vi "Open vi Reference_3.0.0.0.vi"(4 "Close Front Panel(T)":bool, 5 "Wait Until Done":bool=TRUE, 6 "Front Panel State":T1(ring)=enum."Standard", 7 "Auto Dispose Reference":bool, 8 "error in":errorcluster, 10 "vi path":path) -> (0 "error out":errorcluster, 2 "vi reference":refnum<vi>, 3 "hist_rev":string)   [LabVIEW 2018]
uses:
  <vilib>/Utility/error.llb/DialogType.ctl
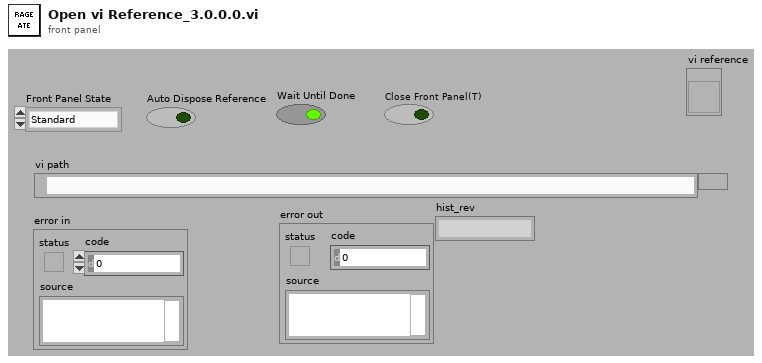
[diagram p1: front panel]
types:
  T1 = enum32{"Invalid", "Standard", "Closed", "Hidden", "Minimized", "Maximized"}
  T2 = typedef "DialogType.ctl" = u16
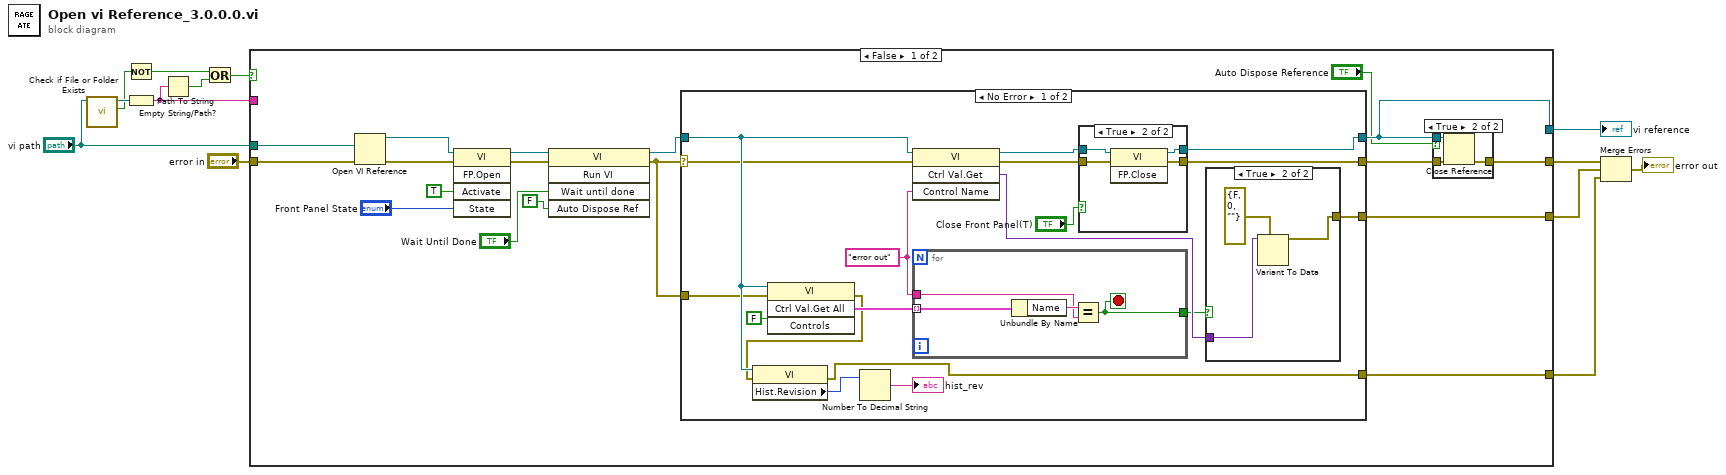
[diagram p0: block diagram]
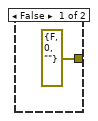
[diagram p3: hidden frame]
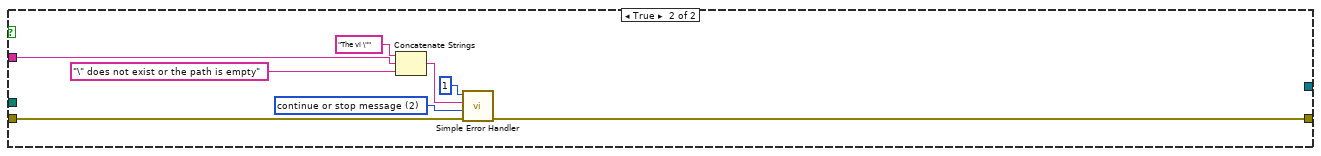
[diagram p6: hidden frame]
diagram:
  n1 = call <vilib>:"Check if File or Folder Exists.vi"("path"="vi path") -> ("file or folder exists?"=w8:bool, "dup path"=w10:path)  [unwired: 8 in, 1 out]
  n2 = Not(x=w8) -> (.not. x?=w5:bool)
  n3 = Path To String(path=w10) -> (string=w9:string)
  n4 = Empty String/Path?(string/path=w9) -> (empty?=w6:bool)
  n5 = Or(x=w5, y=w6) -> (x .or. y?=w7:bool)
  n6 = case shown="False" w7 {
    tunnel: [w17 _] -> w13
    tunnel: "vi path" -> [w31 _]
    tunnel: "error in" -> [w24 w76]
    tunnel: [w18 w70] -> w4
    tunnel: w9 -> [_ w71]
    tunnel: [w22 _] -> w2
    tunnel: [w14 _] -> w1
    frame False {
      n7 = Open VI Reference(vi path=w31, error in (no error)=w24) -> (vi reference=w23:refnum<vi>, error out=w28:errorcluster)  [unwired: 4 in]
      n8 = invoke class="VI" method="FP.Open"(reference=w23, error in=w28, "Activate"=TRUE ("Activate FP?"), "State"="Front Panel State") -> (reference out=w25:refnum<vi>, error out=w27:errorcluster)  [unwired: 1 in, 3 out]
      n9 = invoke class="VI" method="Run VI"(reference=w25, error in=w27, "Wait until done"="Wait Until Done", "Auto Dispose Ref"=FALSE ("Auto Dispose Reference")) -> (reference out=w21:refnum<vi>, error out=w15:errorcluster)  [unwired: 1 in, 3 out]
      n10 = case shown="No Error" w15 {
        selector: w15 -> [w39 w68]
        tunnel: [w53 w69] -> w17
        tunnel: [w51 w68] -> w19
        tunnel: [w49 w68] -> w22
        tunnel: w21 -> [w44 w69]
        tunnel: w15 -> [w38 _]
        tunnel: [w37 _] -> w14
        frame No Error {
          w41 = "error out" ("Control Name")
          n11 = invoke class="VI" method="Ctrl Val.Get All"(reference=w44, error in=w38, "Controls"=FALSE) -> (error out=w36:errorcluster, "Get All Control Values Variant"=w42:cluster{"Name":string, "Variant Data":variant}[])  [unwired: 1 in, 2 out]
          n12 = property class="VI"(reference=w44, error in=w36) -> (error out=w37:errorcluster, "Hist.Revision"=w46:u32)  [unwired: 1 out]
          n13 = Number To Decimal String(number=w46) -> (decimal integer string=→"hist_rev":string)  [unwired: 1 in]
          n14 = invoke class="VI" method="Ctrl Val.Get"(reference=w44, error in=w39, "Control Name"=w41) -> (reference out=w48:refnum<vi>, error out=w47:errorcluster, "Get Control Value Variant"=w50:variant)  [unwired: 1 in, 1 out]
          n15 = for {
            tunnel: w42 -> [w61] mode=indexing
            tunnel: w41 -> [w59]
            tunnel: [w58] -> w40
            stop <- w58 stop-if-true
            n16 = Unbundle By Name(w61) -> ("Name"=w60:string)
            n17 = Equal?(x=w60, y=w59) -> (x = y?=w58:bool)
          }
          n18 = case shown="True" "Close Front Panel(T)" {
            tunnel: [w63 w67] -> w53
            tunnel: w48 -> [w63 w66]
            tunnel: [w62 w65] -> w51
            tunnel: w47 -> [w62 w64]
            frame False {
            }
            frame True {
              n19 = invoke class="VI" method="FP.Close"(reference=w66, error in=w64) -> (reference out=w67:refnum<vi>, error out=w65:errorcluster)  [unwired: 1 in, 1 out]
            }
          }
          n20 = case shown="True" w40 {
            tunnel: w50 -> [_ w57]
            tunnel: [errorcluster {"status"=FALSE, "code"=0, "source"=""} ("type") w55] -> w49
            frame False {
            }
            frame True {
              n21 = Variant To Data(type=errorcluster {"status"=FALSE, "code"=0, "source"=""}, Variant=w57) -> (data=w55:errorcluster)  [unwired: 1 in, 1 out]
            }
          }
        }
        frame Error {
        }
      }
      n22 = case shown="True" "Auto Dispose Reference" {
        tunnel: w19 -> [w32 w35]
        tunnel: [w32 w34] -> w18
        tunnel: w17 -> [_ w33]
        frame False {
        }
        frame True {
          n23 = Close Reference(reference=w33, error in (no error)=w35) -> (error out=w34:errorcluster)
        }
      }
    }
    frame True {
      w77 = T2 2 items=["no dialog", "OK message", "continue or stop message", "OK message + warnings", "continue/stop + warnings"] ("type of dialog (OK msg:1)")
      n24 = Concatenate Strings("The vi \"", w71, "\" does not exist or the path is empty" ("string")) -> (w74:string)
      n25 = call <vilib>:"Simple Error Handler.vi"("error code (no error:0)"=1, "error source (\" \")"=w74, "type of dialog (OK msg:1)"=w77, "error in (no error)"=w76) -> ("error out"=w70:errorcluster)  [unwired: 1 in, 4 out]
    }
  }
  "vi reference" <- w13
  n26 = Merge Errors(w4, w2, w1) -> (→"error out":errorcluster)
